vi "Monitor Current Speed.vi"(8 "error in (no error)":errorcluster, 9 "Y-Axis In":refnum<class "iMotion Controller.lvclass">, 10 "X-Axis In":refnum<class "iMotion Controller.lvclass">, 11 "Stage Data Class":refnum<data-value>) -> (0 "error out":errorcluster, 1 "Y-Axis Out":refnum<class "iMotion Controller.lvclass">, 2 "X-Axis Out":refnum<class "iMotion Controller.lvclass">, 3 "Stage Data Class":refnum<data-value>)   [LabVIEW 2022 SP3, in "XY Stage Process.lvlib" / "XY Stage Process.lvclass"]
uses:
  XY Stage Process.lvclass
  XY Stage Process.lvclass/XY Stage Process.ctl
  6046c730-44da-4461-abcf-74f1f8a9aa6a.vi
  XY Stage Data Class/XY Stage Data Class.lvclass
  XY Stage Data Class/Current Speed.ctl
  Axis Objects/iMotion Controller/iMotion Controller.lvclass
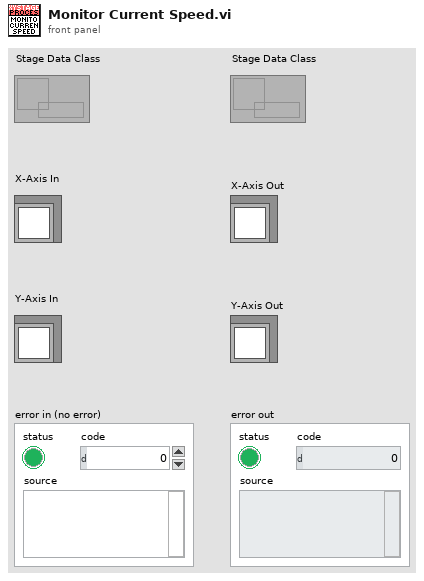
[diagram p1: front panel]
types:
  T1 = typedef "XY Stage Data Class.lvclass/Current Speed.ctl" = cluster{"X Current Speed":dbl, "Y Current Speed":dbl}
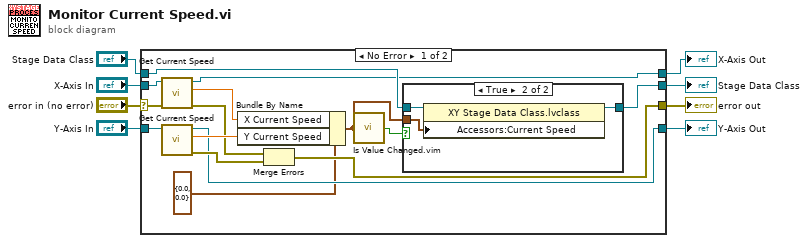
[diagram p0: block diagram]
diagram:
  n1 = case shown="No Error" "error in (no error)" {
    selector: "error in (no error)" -> [w15 w28]
    tunnel: "Y-Axis In" -> [w14 w29]
    tunnel: "X-Axis In" -> [w18 w30]
    tunnel: "Stage Data Class" -> [w22 w31]
    tunnel: [w21 w31] -> w4
    tunnel: [w17 w30] -> w3
    tunnel: [w10 w29] -> w2
    tunnel: [w20 w28] -> w1
    frame No Error {
      n2 = call-dynamic "Get Current Speed.vi"("error in (no error)"=w15, "iMotion Controller in"=w18) -> ("error out"=w11:errorcluster, "Current Speed"=w16:dbl, "iMotion Controller out"=w17:refnum<class "iMotion Controller.lvclass">)  [unwired: 7 in]
      n3 = call-dynamic "Get Current Speed.vi"("iMotion Controller in"=w14) -> ("error out"=w12:errorcluster, "Current Speed"=w13:dbl, "iMotion Controller out"=w10:refnum<class "iMotion Controller.lvclass">)  [unwired: 8 in]
      n4 = Bundle By Name(cluster=T1 {"X Current Speed"=0.0, "Y Current Speed"=0.0} ("Current Speed"), "X Current Speed"=w16, "Y Current Speed"=w13) -> (w19:T1)
      n5 = Merge Errors(w11, w12) -> (w20:errorcluster)
      n6 = call "Is Value Changed.vim"("value"=w19) -> ("changed or first call?"=w23:bool)
      n7 = case shown="True" w23 {
        tunnel: [w24 w27] -> w21
        tunnel: w22 -> [w24 w26]
        tunnel: w19 -> [_ w25]
        frame False {
        }
        frame True {
          n8 = property class="XY Stage Data Class.lvclass"(reference=w26, "Accessors:Current Speed"=w25) -> (reference out=w27:refnum<data-value>)  [unwired: 1 in, 1 out]
        }
      }
    }
    frame Error {
    }
  }
  "Stage Data Class" <- w4
  "X-Axis Out" <- w3
  "Y-Axis Out" <- w2
  "error out" <- w1
